vi "SetUSERCoefficients.vi"(7 "sn":string, 9 "U":dbl[](array[numeric])) -> (2 "output frame":string)   [LabVIEW 2012]
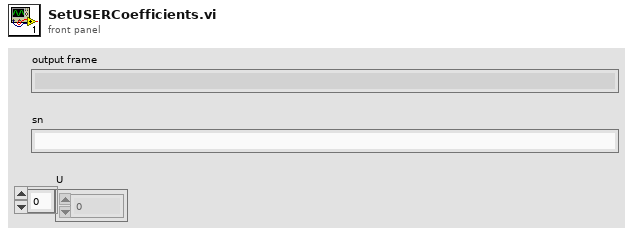
[diagram p1: front panel]
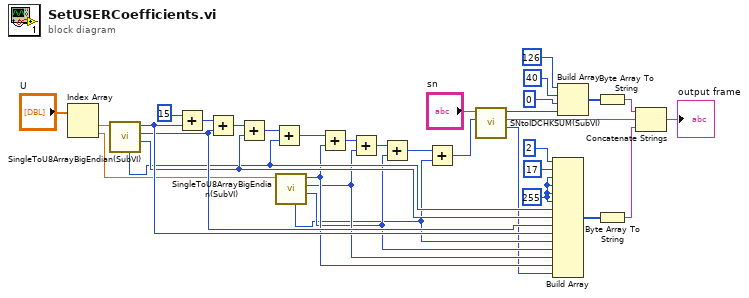
[diagram p0: block diagram]
diagram:
  w33 = u8 255
  n1 = Index Array(array="U") -> (element #1=w4:dbl, element #2=w3:dbl)  [unwired: 2 in]
  n2 = call "SingleToU8ArrayBigEndian(SubVI).vi"("long data"=w4) -> ("third byte"=w16:u8, "send byte"=w19:u8, "first byte"=w20:u8, "forth byte"=w14:u8)  [unwired: 7 in]
  n3 = Add(x=u8 15, y=w20) -> (x+y=w18:u8)
  n4 = Add(x=w18, y=w19) -> (x+y=w17:u8)
  n5 = Add(x=w17, y=w16) -> (x+y=w15:u8)
  n6 = Add(x=w15, y=w14) -> (x+y=w13:u8)
  n7 = call "SingleToU8ArrayBigEndian(SubVI).vi"("long data"=w3) -> ("third byte"=w8:u8, "send byte"=w10:u8, "first byte"=w11:u8, "forth byte"=w6:u8)  [unwired: 7 in]
  n8 = Add(x=w13, y=w11) -> (x+y=w12:u8)
  n9 = Add(x=w12, y=w10) -> (x+y=w9:u8)
  n10 = Add(x=w9, y=w8) -> (x+y=w7:u8)
  n11 = Add(x=w7, y=w6) -> (x+y=w1:u8)
  n12 = call "SNtoIDCHKSUM(SubVI).vi"("fix cheksum"=w1, "input sn"="sn") -> ("output check sum"=w2:u8, "output sn"=w30:string, "output id"=w27:u8)  [unwired: 7 in]
  n13 = Build Array(u8 2, u8 17, w33, w33, w33, w33, w14, w16, w19, w20, w6, w8, w10, w11, w2) -> (w34:u8[])
  n14 = Build Array(u8 126, u8 40, u8 0, w27) -> (w28:u8[])
  n15 = Byte Array To String(unsigned byte array=w28) -> (string=w29:string)
  n16 = Byte Array To String(unsigned byte array=w34) -> (string=w35:string)
  n17 = Concatenate Strings(w29, w30, w35) -> (→"output frame":string)
